vi "Draw Mecanum Wheel.vi"(6 "wheel state":T1, 7 "picture info":T3={"picture size"={"Width"=500, "Height"=500}, "pixels per unit"=10.0}, 8 "error in (no error)":errorcluster, 9 "draw wheel options":T2={"global wheel position"={"x"=0.0, "y"=0.0}, "wheel frame angle (rad)"=0.0, "color (black)"=0, "draw wheel state"=FALSE, "draw forward velocity"=FALSE, "velocity scale"=16711680.0, "velocity color (red)"=16711680}, 10 "picture in":picture, 11 "wheel in":refnum<class "NI_Robotics_Wheel.lvclass">) -> (0 "error out":errorcluster, 2 "picture out":picture, 3 "wheel out":refnum<class "NI_Robotics_Wheel.lvclass">)   [LabVIEW 2017, in "NI_Robotics_Steering Picture.lvlib"]
uses:
  <vilib>/robotics/Utilities/Visualization/Steering Visualization/Steering Picture/NI_Robotics_Steering Picture.lvlib
  <vilib>/robotics/Steering/Wheel/NI_Robotics_Wheel.lvclass
  <vilib>/robotics/Utilities/Visualization/Steering Visualization/Steering Picture/Picture Info.ctl
  <vilib>/Utility/miscctls.llb/LVBoundsTypeDef.ctl
  <vilib>/robotics/Utilities/Visualization/Steering Visualization/Steering Picture/Draw Wheel Options.ctl
  <vilib>/robotics/Steering/Wheel/Wheel State.ctl
  <vilib>/robotics/Steering/Mecanum Wheel/Roller Orientation.ctl
  <vilib>/Analysis/coordinate.llb/2D Cartesian Coordinate Rotation.vi
  <vilib>/Analysis/coordinate.llb/2D Cartesian Coordinate Rotation (Array).vi
  <vilib>/robotics/Utilities/Visualization/Steering Visualization/Steering Picture/Global Position to Pixel.vi
  <vilib>/Analysis/coordinate.llb/Angle Rotation.vi
  <vilib>/Analysis/coordinate.llb/Angle Rotation (scalar).vi
  <vilib>/Analysis/coordinate.llb/Wrap Angle (scalar).vi
  <vilib>/picture/picture.llb/Draw Line.vi
  <vilib>/picture/picture.llb/Move Pen.vi
  <vilib>/picture/picture.llb/Draw Point.vi
  <vilib>/picture/picture.llb/Draw Multiple Lines.vi
  <vilib>/robotics/Steering/Wheel/Get Mecanum Wheel Information.vi
  <vilib>/robotics/Steering/Mecanum Wheel/NI_Robotics_Mecanum Wheel.lvclass
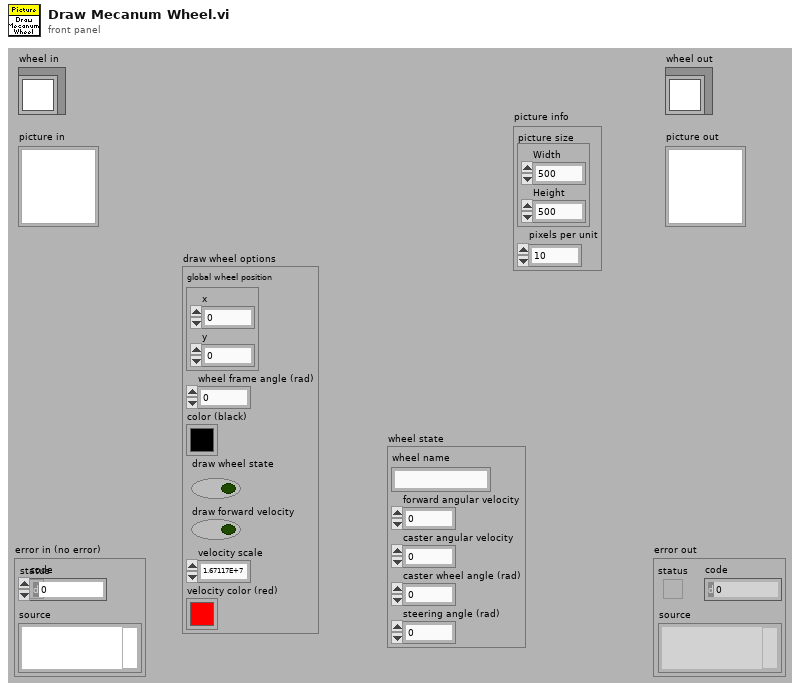
[diagram p1: front panel]
types:
  T1 = typedef "NI_Robotics_Wheel.lvclass/Wheel State.ctl" = cluster{"wheel name":string, "forward angular velocity":dbl, "caster angular velocity":dbl, "caster wheel angle (rad)":dbl, "steering angle (rad)":dbl}
  T2 = typedef "NI_Robotics_Steering Picture.lvlib/Draw Wheel Options.ctl" = cluster{"global wheel position":cluster{"x":dbl, "y":dbl}, "wheel frame angle (rad)":dbl, "color (black)":u32, "draw wheel state":bool, "draw forward velocity":bool, "velocity scale":dbl, "velocity color (red)":u32}
  T3 = typedef "NI_Robotics_Steering Picture.lvlib/Picture Info.ctl" = cluster{"picture size":T4, "pixels per unit":dbl}
  T4 = typedef "LVBoundsTypeDef.ctl" = cluster{"Width":u32, "Height":u32}
  T5 = typedef "NI_Robotics_Mecanum Wheel.lvclass/Roller Orientation.ctl" = u16
  T6 = typedef "NI_Robotics_Wheel.lvclass/Wheel Parameters.ctl" = cluster{"wheel radius":dbl, "gear ratio":dbl, "forward rotation direction":T7}
  T7 = typedef "NI_Robotics_Wheel.lvclass/Rotation Direction.ctl" = u16
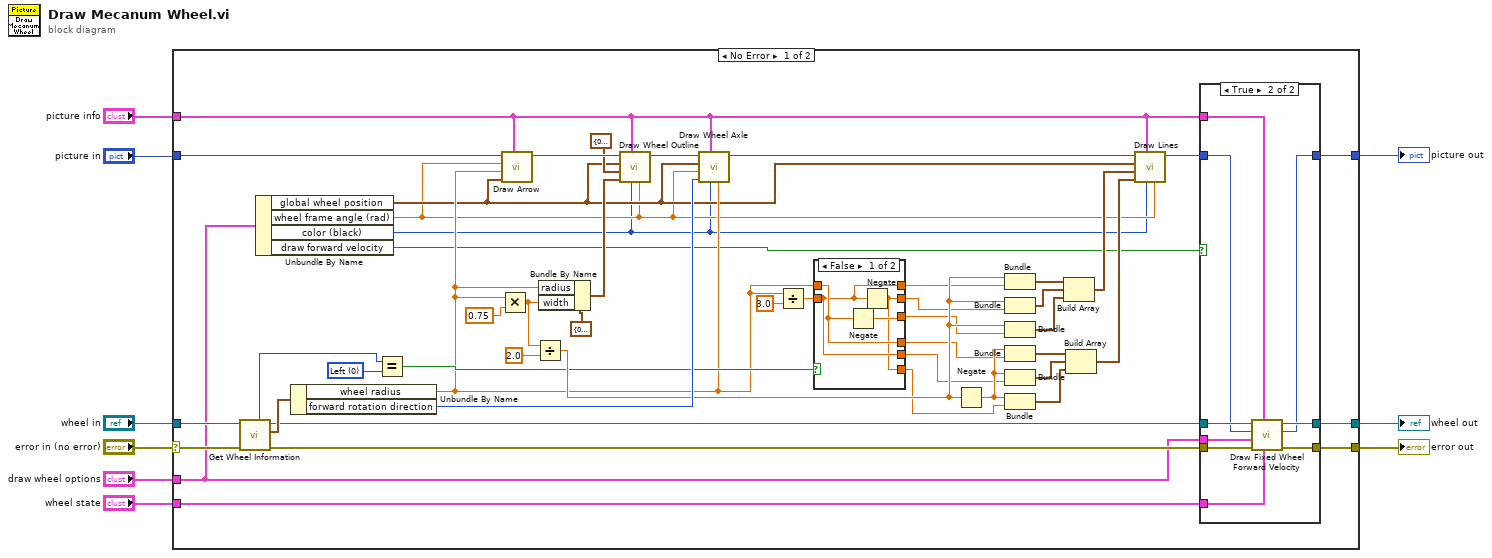
[diagram p0: block diagram]
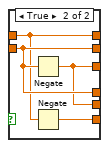
[diagram p3: hidden frame]
diagram:
  n1 = case shown="No Error" "error in (no error)" {
    selector: "error in (no error)" -> [w57 w81]
    tunnel: [w16 w81] -> w5
    tunnel: "wheel in" -> [w58 w79]
    tunnel: "picture in" -> [w55 w80]
    tunnel: [w14 w80] -> w4
    tunnel: [w18 w79] -> w6
    tunnel: "picture info" -> [w13 _]
    tunnel: "draw wheel options" -> [w10 _]
    tunnel: "wheel state" -> [w11 _]
    frame No Error {
      w34 = T5 0 items=["Left", "Right"] ("roller orientation")
      n2 = call-poly <vilib>:"Get Wheel Information.vi"("error in (no error)"=w57, "wheel in"=w58) -> ("error out"=w17:errorcluster, "wheel parameters"=w56:T6, "wheel out"=w19:refnum<class "NI_Robotics_Wheel.lvclass">, "roller orientation"=w33:T5)  [unwired: 4 in, 2 out]
      n3 = Unbundle By Name(w10) -> ("global wheel position"=w22:cluster{"x":dbl, "y":dbl}, "wheel frame angle (rad)"=w21:dbl, "color (black)"=w20:u32, "draw forward velocity"=w12:bool)
      n4 = Unbundle By Name(w56) -> ("wheel radius"=w30:dbl, "forward rotation direction"=w54:T7)
      n5 = Equal?(x=w33, y=w34) -> (x = y?=w31:bool)
      n6 = Multiply(x=w30, y=0.75) -> (x*y=w37:dbl)
      n7 = call <vilib>:"Draw Arrow.vi"("picture info"=w13, "global base position"=w22, "length"=w30, "wheel frame angle (rad)"=w21, "picture in"=w55) -> ("picture out"=w53:picture)  [unwired: 6 in]
      n8 = Divide(x=w37, y=2.0) -> (x/y=w36:dbl)
      n9 = Bundle By Name(cluster=cluster{"radius":dbl, "width":dbl} {"radius"=0.0, "width"=0.0} ("size"), "radius"=w30, "width"=w37) -> (w49:cluster{"radius":dbl, "width":dbl})
      n10 = call <vilib>:"Draw Wheel Outline.vi"("angle (rad)"=w21, "color (black)"=w20, "picture info"=w13, "size"=w49, "offset from center"=cluster{"x":dbl, "y":dbl} {"x"=0.0, "y"=0.0}, "global wheel position"=w22, "picture in"=w53) -> ("picture out"=w52:picture)  [unwired: 4 in]
      n11 = call <vilib>:"Draw Wheel Axle.vi"("length"=w30, "color (black)"=w20, "picture info"=w13, "rotation direction"=w54, "wheel frame angle (rad)"=w21, "global wheel position"=w22, "picture in"=w52) -> ("picture out"=w47:picture)  [unwired: 4 in]
      n12 = Divide(x=w30, y=3.0) -> (x/y=w29:dbl)
      n13 = case shown="False" w31 {
        tunnel: w30 -> [w73 w76]
        tunnel: w29 -> [w72 w78]
        tunnel: [w72 w76] -> w28
        tunnel: [w71 w78] -> w27
        tunnel: [w74 w77] -> w26
        tunnel: [w73 w78] -> w25
        tunnel: [w72 w77] -> w24
        tunnel: [w71 w75] -> w23
        frame False {
          n14 = Negate(x=w73) -> (-x=w74:dbl)
          n15 = Negate(x=w72) -> (-x=w71:dbl)
        }
        frame True {
          n16 = Negate(x=w78) -> (-x=w77:dbl)
          n17 = Negate(x=w76) -> (-x=w75:dbl)
        }
      }
      n18 = Negate(x=w36) -> (-x=w35:dbl)
      n19 = Bundle(w36, "wheel radius"=w28) -> (w41:cluster{dbl, "wheel radius":dbl})  [unwired: 1 in]
      n20 = Bundle(w36, w27) -> (w42:cluster{dbl, dbl})  [unwired: 1 in]
      n21 = Bundle(w36, w26) -> (w43:cluster{dbl, dbl})  [unwired: 1 in]
      n22 = Bundle(w35, "wheel radius"=w25) -> (w44:cluster{dbl, "wheel radius":dbl})  [unwired: 1 in]
      n23 = Bundle(w35, w24) -> (w45:cluster{dbl, dbl})  [unwired: 1 in]
      n24 = Bundle(w35, w23) -> (w46:cluster{dbl, dbl})  [unwired: 1 in]
      n25 = Build Array(w41, w42, w43) -> (w40:cluster{dbl, "wheel radius":dbl}[])
      n26 = Build Array(w44, w45, w46) -> (w39:cluster{dbl, "wheel radius":dbl}[])
      n27 = call <vilib>:"Draw Lines.vi"("wheel frame angle (rad)"=w21, "color (black)"=w20, "picture info"=w13, "end points"=w39, "start points"=w40, "global wheel position"=w22, "picture in"=w47) -> ("picture out"=w15:picture)  [unwired: 4 in]
      n28 = case shown="True" w12 {
        tunnel: w19 -> [w60 w70]
        tunnel: [w60 w69] -> w18
        tunnel: w17 -> [w59 w68]
        tunnel: [w59 w67] -> w16
        tunnel: w15 -> [w61 w66]
        tunnel: [w61 w65] -> w14
        tunnel: w13 -> [_ w64]
        tunnel: w11 -> [_ w63]
        tunnel: w10 -> [_ w62]
        frame False {
        }
        frame True {
          n29 = call <vilib>:"Draw Fixed Wheel Forward Velocity.vi"("wheel state"=w63, "picture info"=w64, "error in (no error)"=w68, "draw wheel options"=w62, "picture in"=w66, "wheel in"=w70) -> ("error out"=w67:errorcluster, "picture out"=w65:picture, "wheel out"=w69:refnum<class "NI_Robotics_Wheel.lvclass">)  [unwired: 3 in]
        }
      }
    }
    frame Error {
    }
  }
  "error out" <- w5
  "wheel out" <- w6
  "picture out" <- w4
